vi "getValuesBool.vi"(8 "error in":errorcluster, 9 "timeout in ms (-1)":i32=100, 11 "notifiers in":refnum<notifier>[](array[refnum])) -> (0 "error out":errorcluster, 2 "notifier values":string[](array[string]), 3 "notifier names":string[](array[string]))   [LabVIEW 2013]
doc: "Takes an array of notifiers and returns two arrays containing the name and value of each notifier. All values have been flattened to strings.\nNotifier value must be a boolean.\n\nKaitlin Gallagher\n3/4/14"
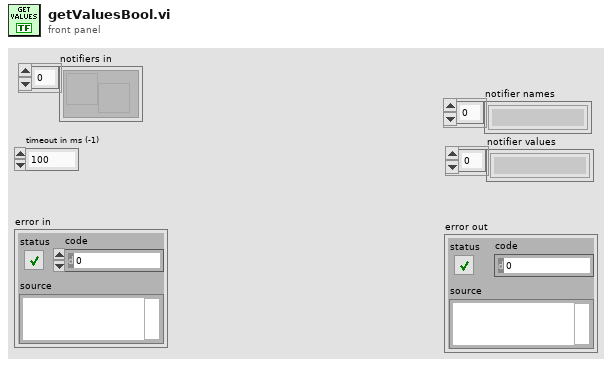
[diagram p1: front panel]
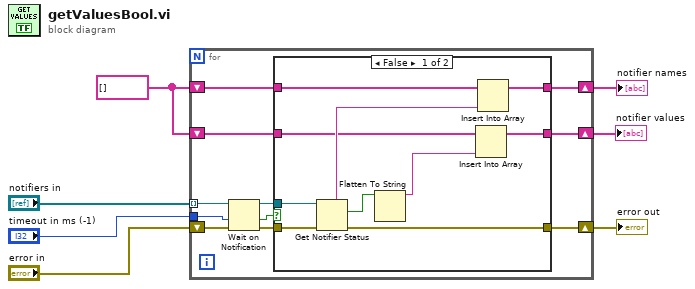
[diagram p0: block diagram]
diagram:
  w4 = string[] [] ("notifier names 2")
  n1 = for {
    shift-right: [w18] -> w6
    shift-left: "error in" -> [w16]
    tunnel: "timeout in ms (-1)" -> [w14]
    shift-right: [w11] -> w2
    shift-left: w4 -> [w12]
    shift-right: [w9] -> w1
    shift-left: w4 -> [w10]
    tunnel: "notifiers in" -> [w8] mode=indexing
    n2 = Wait on Notification(notifier=w8, timeout in ms (-1)=w14, error in (no error)=w16) -> (notifier out=w17:refnum<notifier>, timed out?=w13:bool, error out=w15:errorcluster)  [unwired: 1 in, 1 out]
    n3 = case shown="False" w13 {
      tunnel: [w28 w31] -> w18
      tunnel: w17 -> [w26 _]
      tunnel: w15 -> [w25 w31]
      tunnel: w12 -> [w24 w30]
      tunnel: [w23 w30] -> w11
      tunnel: w10 -> [w20 w29]
      tunnel: [w19 w29] -> w9
      frame False {
        n4 = Get Notifier Status(notifier=w26, error in (no error)=w25) -> (notifier name=w22:string, current notification=w27:bool, error out=w28:errorcluster)  [unwired: 2 out]
        n5 = Flatten To String(anything=w27) -> (data string=w21:string)  [unwired: 3 in, 2 out]
        n6 = Insert Into Array(array=w20, new element=w21) -> (w19:string[])  [unwired: 1 in]
        n7 = Insert Into Array(array=w24, new element=w22) -> (w23:string[])  [unwired: 1 in]
      }
      frame True {
      }
    }
  }
  "error out" <- w6
  "notifier names" <- w2
  "notifier values" <- w1
